vi "InsertNewItem.vi"(7 "Replace?":bool, 8 "error in (no error)":errorcluster, 9 "IDependencyRule in":refnum<class "IDependencyItemRule.lvclass">, 11 "CRuleList in":refnum<class "CRuleList.lvclass">) -> (0 "error out":errorcluster, 2 "New key?":bool, 3 "CRuleList out":refnum<class "CRuleList.lvclass">)   [LabVIEW 2020, in "DependencyInspection.lvlib" / "CRuleList.lvclass"]
uses:
  CRuleList.lvclass
  <vilib>/Utility/miscctls.llb/LVMapReplaceAction.ctl
  LabVIEWObjectInterfaces/IDependencyItemRule/IDependencyItemRule.lvclass
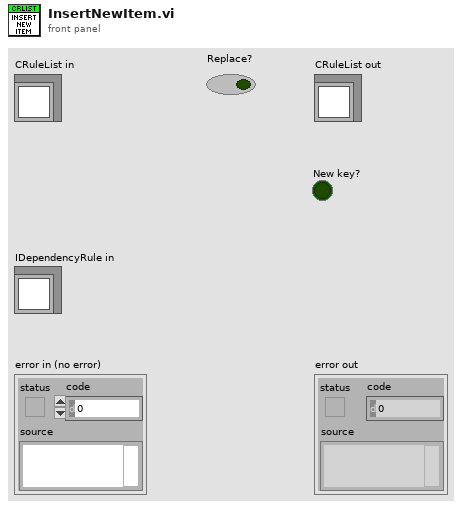
[diagram p1: front panel]
types:
  T1 = typedef "LVMapReplaceAction.ctl" = enum32{"Modify Entry only if found", "Add or Modify Entry", "Delete Entry"}
  T2 = typedef "DependencyInspection.lvlib/CRuleList.lvclass/RuleListRef.ctl" = refnum<data-value>
  T3 = typedef "DependencyInspection.lvlib/CRuleList.lvclass/RuleList.ctl" = map{string, refnum<class "IDependencyItemRule.lvclass">}
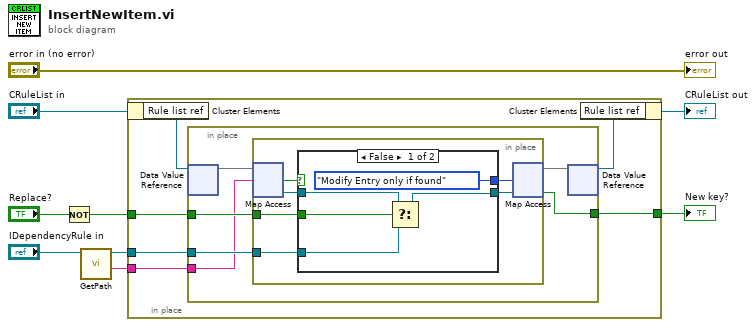
[diagram p0: block diagram]
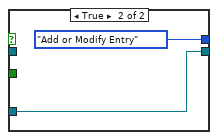
[diagram p2: hidden frame]
diagram:
  n1 = Not(x="Replace?") -> (.not. x?=w2:bool)
  n2 = call-dynamic "GetPath.vi"("ILabVIEWItem in"="IDependencyRule in") -> ("Path"=w1:string, "ILabVIEWItem out"=w8:refnum<class "IDependencyItemRule.lvclass">)  [unwired: 8 in, 1 out]
  n3 = in-place {
    in-place-border: w1 -> [w12]
    in-place-border: w8 -> [w15]
    in-place-border: [w14] -> w4
    in-place-border: w2 -> [w13]
    n4 = in-place-cluster #1("CRuleList in") -> ("Rule list ref"=w11:T2)
    n5 = in-place {
      in-place-border: w15 -> [w21]
      in-place-border: [w20] -> w14
      in-place-border: w13 -> [w19]
      in-place-border: w12 -> [w18]
      n6 = in-place-dvr #2(w11) -> (w17:T3)  [unwired: 1 out]
      n7 = in-place {
        in-place-border: w21 -> [w23]
        in-place-border: w19 -> [w22]
        n8 = in-place-map #3(w17, w18) -> (w24:refnum<class "IDependencyItemRule.lvclass">, w27:bool)  [unwired: 1 in]
        n9 = case shown="False" w27 {
          tunnel: [LVMapReplaceAction."Modify Entry only if found" ("action") LVMapReplaceAction."Add or Modify Entry" ("action")] -> w26
          tunnel: [w29 w33] -> w25
          tunnel: w24 -> [w30 _]
          tunnel: w23 -> [w28 w33]
          tunnel: w22 -> [w31 _]
          frame False {
            n10 = Select(t=w30, s=w31, f=w28) -> (s? t:f=w29:refnum<class "IDependencyItemRule.lvclass">)
          }
          frame True {
          }
        }
        n11 = in-place-map #3(w25, w26) -> (w16:T3, w20:bool)  [unwired: 1 out]
      }
      n12 = in-place-dvr #2(w16) -> (w10:T2)  [unwired: 1 out]
    }
    n13 = in-place-cluster #1("Rule list ref"=w10) -> (→"CRuleList out":refnum<class "CRuleList.lvclass">)
  }
  "New key?" <- w4
  "error out" <- "error in (no error)"
